vi "BuildCallFunction.vi"(1 "StatementName":string, 2 "ParameterNum":u16) -> (0 "StatementText":string)   [LabVIEW 2011]
doc: "Construct the procedure: {call ------- (?,?...)}"
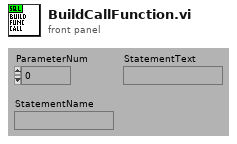
[diagram p1: front panel]
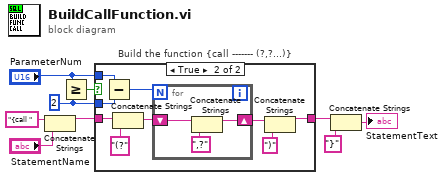
[diagram p0: block diagram]
diagram:
  w9 = u16 2 ("x")
  n1 = Concatenate Strings("{call ", "StatementName") -> (w5:string)
  n2 = Greater Or Equal?(x="ParameterNum", y=w9) -> (x >= y?=w2:bool)
  n3 = case "Build the function {call ------- (?,?...)}" shown="True" w2 {
    tunnel: w5 -> [w10 w19]
    tunnel: [w10 w16] -> w6
    tunnel: "ParameterNum" -> [_ w15]
    tunnel: w9 -> [_ w11]
    frame False {
    }
    frame True {
      n4 = Subtract(x=w15, y=w11) -> (x-y=w14:u16)
      n5 = Concatenate Strings(w19, "(?") -> (w13:string)
      n6 = for {
        N: w14 -> [_]
        shift-right: [w20] -> w12
        shift-left: w13 -> [w21]
        n7 = Concatenate Strings(w21, ",?") -> (w20:string)
      }
      n8 = Concatenate Strings(w12, ")") -> (w16:string)
    }
  }
  n9 = Concatenate Strings(w6, "}") -> (→"StatementText":string)
